vi "XY Graph [0-1]-Normalize Plot.vi"(8 "error in (no error)":errorcluster, 9 "Replace Plot (T)?":bool=TRUE, 11 "Selected Plot Info":T1={"Multiplot XY Graph"=refnum, "Mouse Coordinates"={"Horizontal"=0, "Vertical"=0}, "Plot Index"=-1}) -> (0 "Error Out":errorcluster, 1 "[0-1]-Normalize Plot Message":string, 3 "[0-1]-Normalized Plot":cluster{"t Array":dbl[], "IRF Array":dbl[]})   [LabVIEW 2021, in "XY Graph Add-Ons.lvlib"]
uses:
  XY Graph Add-Ons.lvlib
  XY Graph Selected Plot Info.ctl
  XY Graph Refnum.ctl
  <vilib>/Utility/miscctls.llb/LVPoint32TypeDef.ctl
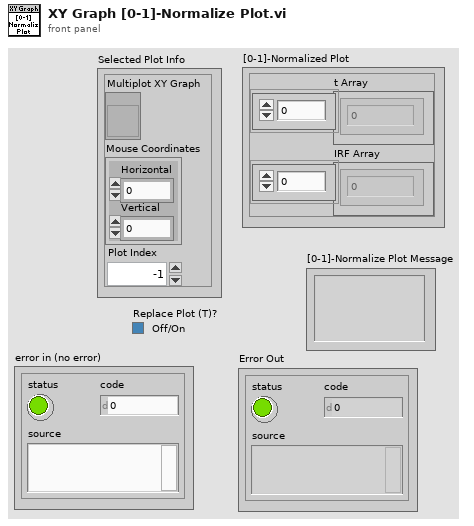
[diagram p1: front panel]
types:
  T1 = typedef "XY Graph Add-Ons.lvlib/XY Graph Selected Plot Info.ctl" = cluster{"Multiplot XY Graph":T2, "Mouse Coordinates":T3, "Plot Index":i32}
  T2 = typedef "XY Graph Add-Ons.lvlib/XY Graph Refnum.ctl" = refnum<vi>
  T3 = typedef "LVPoint32TypeDef.ctl" = cluster{"Horizontal":i32, "Vertical":i32}
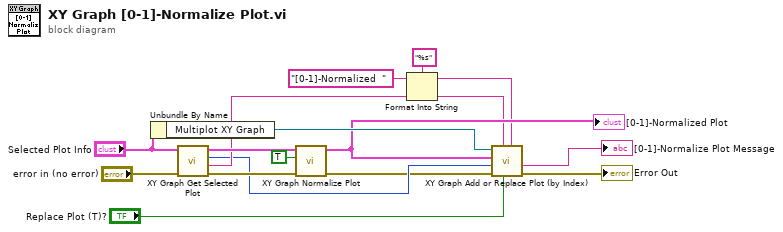
[diagram p0: block diagram]
diagram:
  n1 = Unbundle By Name("Selected Plot Info") -> ("Multiplot XY Graph"=w9:T2)
  n2 = call "XY Graph Get Selected Plot.vi"("error in (no error)"="error in (no error)", "Selected Plot Info"="Selected Plot Info") -> ("error out"=w11:errorcluster, "Plot Name"=w6:string, "Plot Index"=w4:i32, "Plot"=w12:cluster{"X Array":dbl[], "Y Array":dbl[]})  [unwired: 4 in, 2 out]
  n3 = call "XY Graph Normalize Plot.vi"("Error In"=w11, "Subtract Baseline? (No)"=TRUE, "Plot in"=w12) -> ("Error Out"=w3:errorcluster, "Plot out"=w8:cluster{"X Array":dbl[], "Y Array":dbl[]})  [unwired: 7 in]
  "[0-1]-Normalized Plot" <- w8
  n4 = Format Into String(format string="%s", initial string="[0-1]-Normalized  ", w6) -> (resulting string=w5:string)  [unwired: 1 in, 1 out]
  n5 = call "XY Graph Add or Replace Plot (by Index).vi"("New Plot Name"=w5, "Replace Plot (T)?"="Replace Plot (T)?", "Original Plot Name"=w6, "error in (no error)"=w3, "Plot Index"=w4, "Plot in"=w8, "XYGraph in"=w9) -> ("error out"=→"Error Out":errorcluster, "Message"=→"[0-1]-Normalize Plot Message":string)  [unwired: 3 in]
